vi "PS_Waveform_Chart.vi"(1 "stop":bool, 2 "SCPI":T1 items=["*IDN?", "*SAV 1", "*RCL 1", "INSTTrument CH1", "INSTTrument CH2", "INSTrument?", "MEASure:CURRent? CH1", "MEASure:CURRent? CH2", "MEASure:VOLTage? CH1", "MEASure:VOLTage? CH2", "MEASure:POWEr? CH1", "MEASure:POWEr? CH2", "CH1:CURRent?", "CH2:CURRent?", "CH1:VOLTage? ", "CH2:VOLTage? ", "OUTPut CH1,ON", "OUTPut CH1,OFF", "OUTPut CH2,ON", "OUTPut CH2,OFF", "OUTPut CH3,ON", "OUTPut CH3,OFF", "OUTPut:TRACK 0", "OUTPut:TRACK 1", "OUTPut:TRACK 2", "OUTPut:WAVE CH1,ON", "OUTPut:WAVE CH1,OFF", "OUTPut:WAVE CH2,ON", "OUTPut:WAVE CH2,OFF"], 3 "VISA":refnum<visa-resource-name>) -> (0 "Waveform Chart":dbl(graph))   [LabVIEW 2020]
doc: "Reading value from PS and paint on Waveform Chart"
uses:
  controls/SCPI_enum.ctl
  <vilib>/Utility/file.llb/Write Delimited Spreadsheet (DBL).vi
panel:
  in  "file path (dialog if empty)":path
  out "value":dbl
  out "read buffer":string
  out "error out":errorcluster
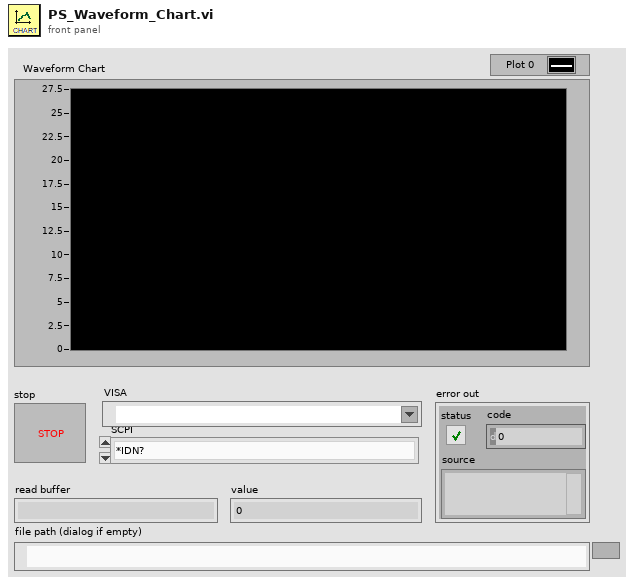
[diagram p1: front panel]
types:
  T1 = typedef "SCPI_enum.ctl" = u16
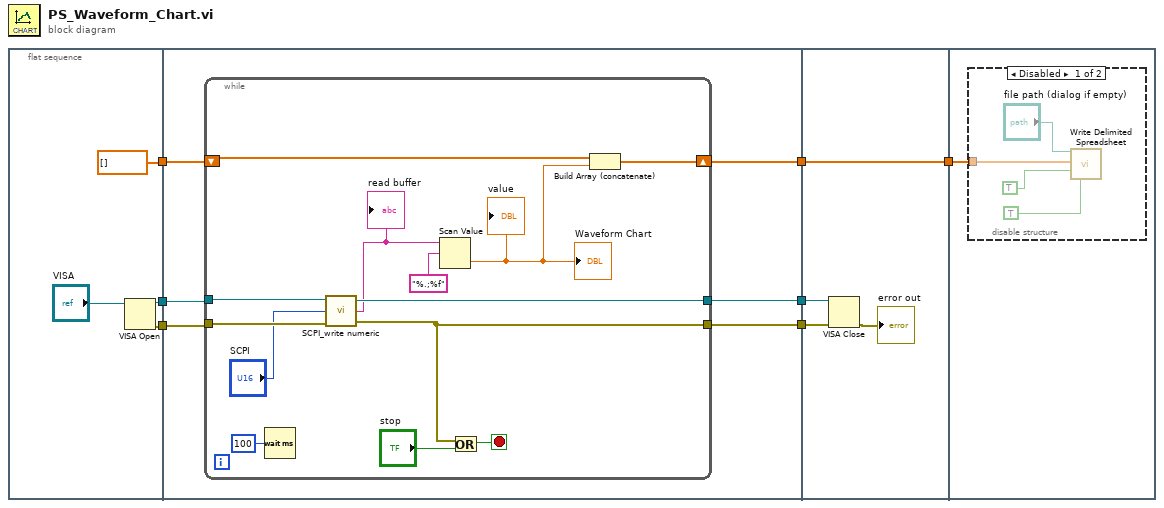
[diagram p0: block diagram]
diagram:
  n1 = flat-sequence {
    tunnel: [dbl[] []] -> w7
    tunnel: [w10] -> w6
    tunnel: [w9] -> w5
    tunnel: w7 -> [w15]
    tunnel: w6 -> [w13]
    tunnel: w5 -> [w12]
    tunnel: [w17] -> w4
    tunnel: [w16] -> w3
    tunnel: [w14] -> w2
    tunnel: w4 -> [w32]
    tunnel: w3 -> [w31]
    tunnel: w2 -> [w34]
    tunnel: [w34] -> w1
    tunnel: w1 -> [w35]
    frame #0 {
      n2 = VISA Open(VISA resource name="VISA") -> (VISA resource name=w9:refnum<visa-resource-name>, error out=w10:errorcluster)  [unwired: 4 in]
    }
    frame #1 {
      n3 = while {
        tunnel: [w28] -> w17
        tunnel: w12 -> [w27]
        tunnel: w13 -> [w26]
        tunnel: [w25] -> w16
        shift-right: [w18] -> w14
        shift-left: w15 -> [w19]
        stop <- w29 stop-if-true
        n4 = Wait (ms)(milliseconds to wait=u32 100) -> ()  [unwired: 1 out]
        n5 = call "SCPI_write numeric.vi"("error in (no error)"=w26, "SCIPI"="SCPI", "VISA"=w27) -> ("error out"=w28:errorcluster, "read buffer"=w24:string, "VISA resource name out"=w25:refnum<visa-resource-name>)
        "read buffer" <- w24
        n6 = Scan Value(string=w24, format string="%.;%f") -> (value=w20:dbl)  [unwired: 1 in, 1 out]
        "Waveform Chart" <- w20
        "value" <- w20
        n7 = Or(x=w28, y="stop") -> (x .or. y?=w29:bool)
        n8 = Build Array (concatenate)(w19, w20) -> (w18:dbl[])
      }
    }
    frame #2 {
      n9 = VISA Close(VISA resource name=w31, error in (no error)=w32) -> (error out=→"error out":errorcluster)
    }
    frame #3 {
      n10 = disable-structure shown="Disabled" {
        disable-tunnel: w35 -> [w38 _]
        frame Disabled {
          n11 = call-poly <vilib>:"Write Delimited Spreadsheet.vi"("file path (dialog if empty)"="file path (dialog if empty)", "1D data"=w38, "append to file? (new file:F)"=TRUE, "transpose? (no:F)"=TRUE) -> ()  [unwired: 10 in, 2 out]
        }
        frame Enabled {
        }
      }
    }
  }
